vi "CH_LM App Windows.vi"(0 "Option":string) -> ()   [LabVIEW 2012, in "CH_LM App.lvlib"]
doc: "This VI is used to organize Child windows on the desktop."
uses:
  CH_LM App.lvlib
panel:
  in  "Window Bounds":T1
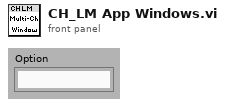
[diagram p1: front panel]
types:
  T1 = cluster{"left":i16, "top":i16, "right":i16, "bottom":i16}
  T2 = typedef "LVRectTypeDef.ctl" = cluster{"Left":i16, "Top":i16, "Right":i16, "Bottom":i16}
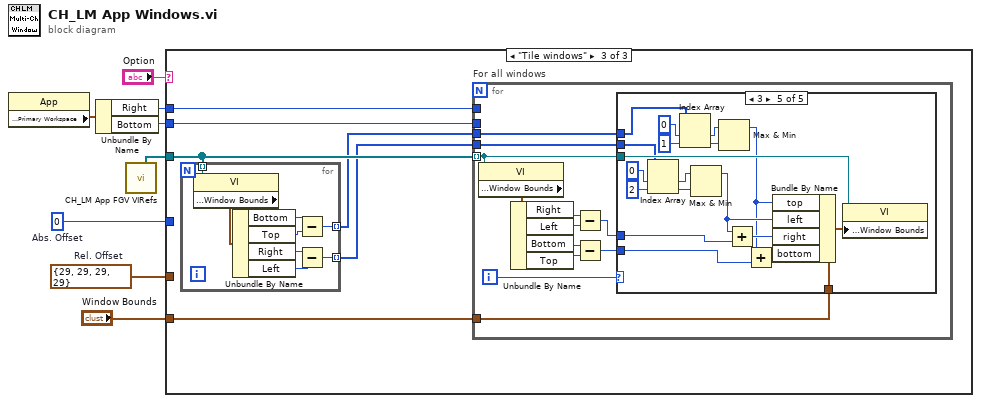
[diagram p0: block diagram]
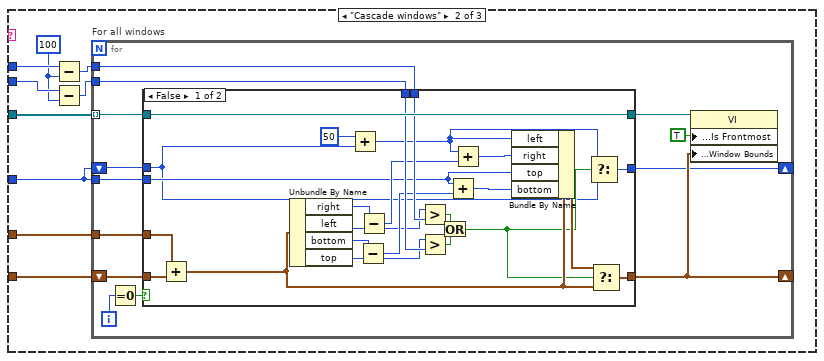
[diagram p3: hidden frame]
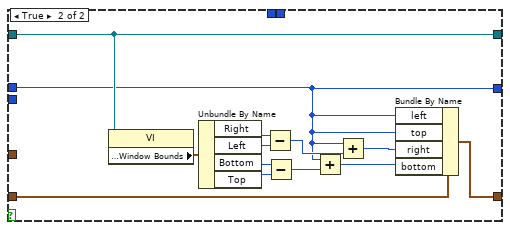
[diagram p4: hidden frame]
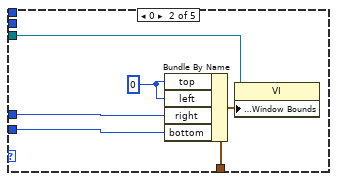
[diagram p6: hidden frame]
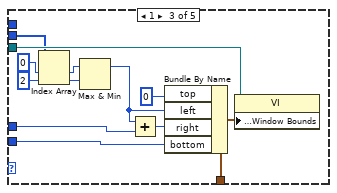
[diagram p7: hidden frame]
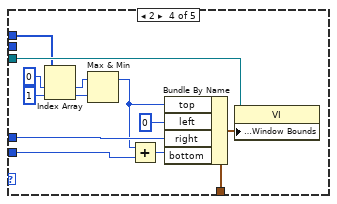
[diagram p8: hidden frame]
diagram:
  w2 = T1 {"left"=29, "top"=29, "right"=29, "bottom"=29}  # Rel. Offset
  w3 = i16 0  # Abs. Offset
  n1 = property on="Property Node" class="App"() -> ("Display:Primary Workspace"=w8:T2)  [unwired: 2 in, 2 out]
  n2 = Unbundle By Name(w8) -> ("Right"=w6:i16, "Bottom"=w5:i16)
  n3 = call "CH_LM App FGV VIRefs.vi"() -> ("VI Refs"=w1:refnum<vi>[])  [unwired: 4 in, 7 out]
  n4 = case shown="\"Tile windows\"" "Option" {
    tunnel: w1 -> [_ w17 w70]
    tunnel: w6 -> [_ w12 w73]
    tunnel: w5 -> [_ w10 w72]
    tunnel: "Window Bounds" -> [_ w16 w71]
    tunnel: w2 -> [_ w15 _]
    tunnel: w3 -> [_ w14 _]
    frame Default {
    }
    frame "Cascade windows" {
      w9 = i16 100 ("x")
      n5 = Subtract(x=w12, y=w9) -> (x-y=w13:i16)
      n6 = Subtract(x=w10, y=w9) -> (x-y=w11:i16)
      n7 = for "For all windows" {
        tunnel: w13 -> [w29]
        tunnel: w11 -> [w30]
        tunnel: w17 -> [w24] mode=indexing
        shift-right: [w22] -> _
        shift-left: w16 -> [w28]
        tunnel: w15 -> [w25]
        shift-right: [w19] -> _
        shift-left: w14 -> [w20]
        tunnel: w14 -> [w18]
        i -> [w26]
        n8 = Equal To 0?(x=w26) -> (x = 0?=w27:bool)
        n9 = case shown="False" w27 {
          tunnel: w30 -> [w50 _]
          tunnel: w29 -> [w51 _]
          tunnel: w24 -> [w52 w56]
          tunnel: w28 -> [w54 w62]
          tunnel: [w44 w61] -> w22
          tunnel: w25 -> [w53 _]
          tunnel: [w52 w56] -> w23
          tunnel: w20 -> [w33 w55]
          tunnel: [w35 w55] -> w19
          tunnel: w18 -> [w38 _]
          frame False {
            n10 = Add(x=w53, y=w54) -> (x+y=w45:T1)
            n11 = Unbundle By Name(w45) -> ("right"=w47:i16, "left"=w32:i16, "bottom"=w46:i16, "top"=w31:i16)
            n12 = Add(x=i16 50, y=w33) -> (x+y=w36:i16)
            n13 = Subtract(x=w46, y=w31) -> (x-y=w40:i16)
            n14 = Subtract(x=w47, y=w32) -> (x-y=w43:i16)
            n15 = Greater?(x=w32, y=w51) -> (0:w48:bool)
            n16 = Greater?(x=w31, y=w50) -> (0:w49:bool)
            n17 = Or(x=w48, y=w49) -> (x .or. y?=w34:bool)
            n18 = Add(x=w38, y=w40) -> (x+y=w42:i16)
            n19 = Add(x=w36, y=w43) -> (x+y=w41:i16)
            n20 = Bundle By Name(cluster=w45, "left"=w36, "right"=w41, "top"=w38, "bottom"=w42) -> (w37:T1)
            n21 = Select(t=w36, s=w34, f=w33) -> (s? t:f=w35:i16)
            n22 = Select(t=w37, s=w34, f=w45) -> (s? t:f=w44:T1)
          }
          frame True {
            n23 = property class="VI"(reference=w56) -> ("Front Panel Window:Window Bounds"=w63:T2)  [unwired: 1 in, 2 out]
            n24 = Unbundle By Name(w63) -> ("Right"=w66:i16, "Left"=w67:i16, "Bottom"=w65:i16, "Top"=w64:i16)
            n25 = Subtract(x=w66, y=w67) -> (x-y=w59:i16)
            n26 = Subtract(x=w65, y=w64) -> (x-y=w57:i16)
            n27 = Add(x=w55, y=w57) -> (x+y=w58:i16)
            n28 = Add(x=w55, y=w59) -> (x+y=w60:i16)
            n29 = Bundle By Name(cluster=w62, "left"=w55, "top"=w55, "right"=w60, "bottom"=w58) -> (w61:T1)
          }
        }
        n30 = property class="VI"(reference=w23, "Front Panel Window:Is Frontmost"=TRUE, "Front Panel Window:Window Bounds"=w22) -> ()  [unwired: 1 in, 2 out]
      }
    }
    frame "Tile windows" {
      n31 = for {
        tunnel: w70 -> [w81] mode=indexing
        tunnel: [w75] -> w69 mode=indexing
        tunnel: [w74] -> w68 mode=indexing
        n32 = property class="VI"(reference=w81) -> ("Front Panel Window:Window Bounds"=w76:T2)  [unwired: 1 in, 2 out]
        n33 = Unbundle By Name(w76) -> ("Bottom"=w77:i16, "Top"=w78:i16, "Right"=w80:i16, "Left"=w79:i16)
        n34 = Subtract(x=w77, y=w78) -> (x-y=w75:i16)
        n35 = Subtract(x=w80, y=w79) -> (x-y=w74:i16)
      }
      n36 = for "For all windows" {
        tunnel: w73 -> [_]
        tunnel: w72 -> [_]
        tunnel: w70 -> [w91] mode=indexing
        tunnel: w71 -> [w93]
        tunnel: w69 -> [w82]
        tunnel: w68 -> [w83]
        i -> [w92]
        n37 = property class="VI"(reference=w91) -> ("Front Panel Window:Window Bounds"=w90:T2)  [unwired: 1 in, 2 out]
        n38 = Unbundle By Name(w90) -> ("Right"=w89:i16, "Left"=w88:i16, "Bottom"=w87:i16, "Top"=w86:i16)
        n39 = Subtract(x=w89, y=w88) -> (x-y=w85:i16)
        n40 = Subtract(x=w87, y=w86) -> (x-y=w84:i16)
        n41 = case shown="3" w92 {
          tunnel: w91 -> [_ w99 w112 w125 w144]
          tunnel: w93 -> [_ w97 w110 w123 w142]
          tunnel: w85 -> [_ w95 w106 w121 w140]
          tunnel: w84 -> [_ w94 w108 w119 w138]
          tunnel: w83 -> [_ _ w103 _ w133]
          tunnel: w82 -> [_ _ _ w118 w127]
          frame Default {
          }
          frame 0 {
            w96 = i16 0 ("left")
            n42 = Bundle By Name(cluster=w97, "top"=w96, "left"=w96, "right"=w95, "bottom"=w94) -> (w98:T1)
            n43 = property class="VI"(reference=w99, "Front Panel Window:Window Bounds"=w98) -> ()  [unwired: 1 in, 2 out]
          }
          frame 1 {
            n44 = Index Array(array=w103, index #1=0 ("index"), index #2=2 ("index")) -> (element #1=w101:i16, element #2=w102:i16)
            n45 = Max & Min(x=w101, y=w102) -> (max(x,y)=w100:i16)  [unwired: 1 out]
            n46 = Add(x=w100, y=w106) -> (x+y=w107:i16)
            n47 = Bundle By Name(cluster=w110, "top"=i16 0 ("left"), "left"=w100, "right"=w107, "bottom"=w108) -> (w111:T1)
            n48 = property class="VI"(reference=w112, "Front Panel Window:Window Bounds"=w111) -> ()  [unwired: 1 in, 2 out]
          }
          frame 2 {
            n49 = Index Array(array=w118, index #1=0 ("index"), index #2=1 ("index")) -> (element #1=w114:i16, element #2=w115:i16)
            n50 = Max & Min(x=w114, y=w115) -> (max(x,y)=w113:i16)  [unwired: 1 out]
            n51 = Add(x=w113, y=w119) -> (x+y=w120:i16)
            n52 = Bundle By Name(cluster=w123, "top"=w113, "left"=i16 0, "right"=w121, "bottom"=w120) -> (w124:T1)
            n53 = property class="VI"(reference=w125, "Front Panel Window:Window Bounds"=w124) -> ()  [unwired: 1 in, 2 out]
          }
          frame 3 {
            n54 = Index Array(array=w133, index #1=0 ("index"), index #2=2 ("index")) -> (element #1=w134:i16, element #2=w135:i16)
            n55 = Index Array(array=w127, index #1=0 ("index"), index #2=1 ("index")) -> (element #1=w131:i16, element #2=w130:i16)
            n56 = Max & Min(x=w134, y=w135) -> (max(x,y)=w132:i16)  [unwired: 1 out]
            n57 = Max & Min(x=w131, y=w130) -> (max(x,y)=w126:i16)  [unwired: 1 out]
            n58 = Add(x=w132, y=w140) -> (x+y=w141:i16)
            n59 = Add(x=w126, y=w138) -> (x+y=w139:i16)
            n60 = Bundle By Name(cluster=w142, "top"=w126, "left"=w132, "right"=w141, "bottom"=w139) -> (w143:T1)
            n61 = property class="VI"(reference=w144, "Front Panel Window:Window Bounds"=w143) -> ()  [unwired: 1 in, 2 out]
          }
        }
      }
    }
  }
